vi "Pareto Moments.vi"(9 "c":dbl=3.0, 10 "a":dbl=1.0) -> (0 "error":i32, 2 "variance":dbl=0.75, 3 "mean":dbl=1.5)   [LabVIEW 2018, in "NI_Gmath.lvlib"]
doc: "Returns the expected mean and variance of the random variate X, where X describes the selected distribution type. You must manually select the polymorphic instance to use."
uses:
  NI_Gmath.lvlib
  st_error_code.ctl
panel:
  # "Pareto Moments"
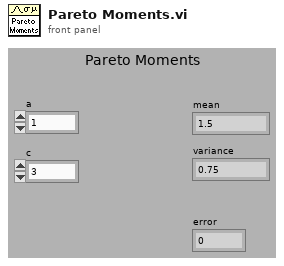
[diagram p1: front panel]
types:
  T1 = typedef "NI_Gmath.lvlib/st_error_code.ctl" = i32
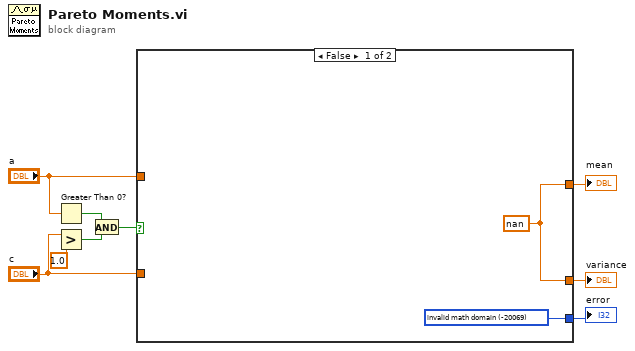
[diagram p0: block diagram]
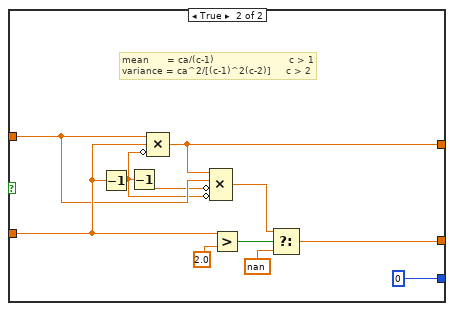
[diagram p2: hidden frame]
diagram:
  n1 = Greater Than 0?(x="a") -> (x > 0?=w4:bool)
  n2 = Greater?(x="c", y=1.0) -> (0:w1:bool)
  n3 = And(x=w4, y=w1) -> (x .and. y?=w9:bool)
  n4 = case shown="False" w9 {
    tunnel: [w11 0 ("invalid math domain")] -> w6
    tunnel: [w10 w18] -> w7
    tunnel: [w10 w12] -> w8
    tunnel: "c" -> [_ w19]
    tunnel: "a" -> [_ w17]
    frame False {
      w11 = T1 -20069 items=["invalid math domain"=-20069, "Fourier interpolation size m >= n"=-20070, "empty array"=-20003] ("stat interp error code")
      w10 = nan
    }
    frame True {
      # "mean      = ca/(c-1)                         c > 1\nvariance = ca^2/[(c-1)^2(c-2)]     c > 2"
      n5 = Decrement(x=w19) -> (x-1=w15:dbl)
      n6 = Decrement(x=w15) -> (x-1=w16:dbl)
      n7 = Compound Arithmetic op=MULTIPLY(w17, w19, invert w15) -> (w18:dbl)
      n8 = Compound Arithmetic op=MULTIPLY(w18, w17, invert w16, invert w15) -> (w14:dbl)
      n9 = Greater?(x=w19, y=2.0) -> (0:w20:bool)
      n10 = Select(t=w14, s=w20, f=nan ("y")) -> (s? t:f=w12:dbl)
    }
  }
  "mean" <- w7
  "error" <- w6
  "variance" <- w8
